vi "Attach Node.vi"(0 "TREE in":refnum<class "MyTreeAPI.lvclass">, 5 "Parent Node":string, 7 "Node ID":string, 9 "Node Name":string, 11 "error in (no error)":errorcluster, 12 "Symbol Index":i32) -> (4 "TREE out":refnum<class "MyTreeAPI.lvclass">, 6 "Node ID":string, 15 "error out":errorcluster)   [LabVIEW 2015, in "MyTreeAPI.lvclass"]
uses:
  MyTreeAPI.lvclass
  MyTreeAPI.lvclass/MyTreeAPI.ctl
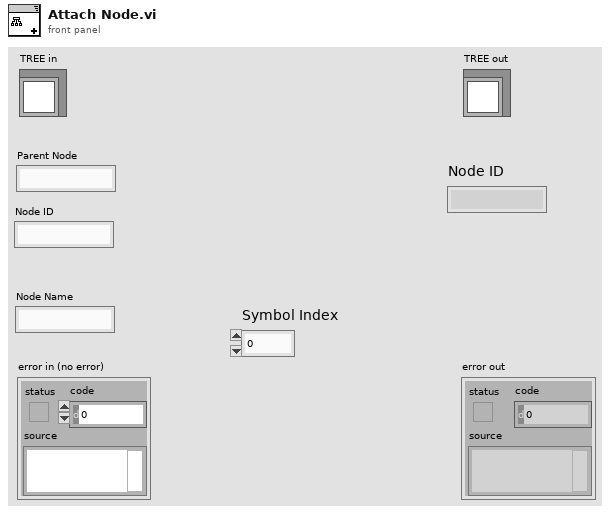
[diagram p1: front panel]
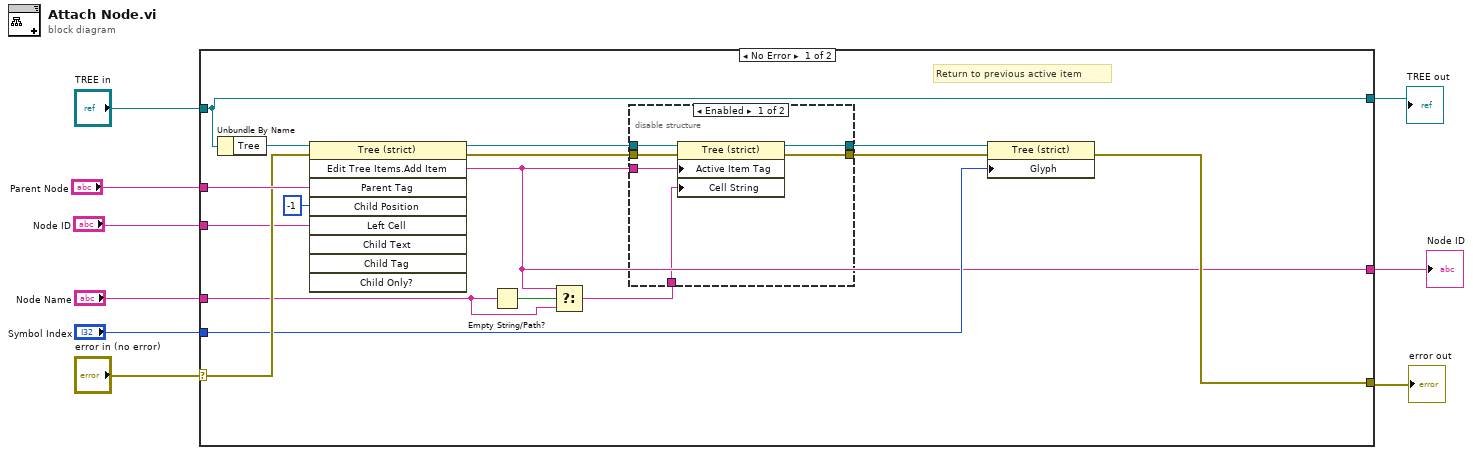
[diagram p0: block diagram]
diagram:
  n1 = case shown="No Error" "error in (no error)" {
    selector: "error in (no error)" -> [w21 w35]
    tunnel: [w19 w35] -> w8
    tunnel: [w25 w34] -> w6
    tunnel: "TREE in" -> [w25 w34]
    tunnel: "Parent Node" -> [w22 _]
    tunnel: "Symbol Index" -> [w20 _]
    tunnel: "Node ID" -> [w18 _]
    tunnel: "Node Name" -> [w13 _]
    tunnel: [w14 _] -> w1
    frame No Error {
      # "Return to previous active item"
      n2 = Unbundle By Name(w25) -> ("Tree"=w23:refnum<vi>)
      n3 = invoke class="Tree (strict)" method="Edit Tree Items.Add Item"(reference=w23, error in=w21, "Parent Tag"=w22, "Child Position"=-1, "Left Cell"=w18) -> (reference out=w17:refnum<vi>, error out=w16:errorcluster, "Edit Tree Items:Add Item"=w14:string)  [unwired: 4 in, 6 out]
      n4 = Empty String/Path?(string/path=w13) -> (empty?=w15:bool)
      n5 = Select(t=w14, s=w15, f=w13) -> (s? t:f=w12:string)
      n6 = disable-structure shown="Enabled" {
        disable-tunnel: w17 -> [w29 w33]
        disable-tunnel: w16 -> [w28 w32]
        disable-tunnel: [w31 w33] -> w11
        disable-tunnel: [w30 w32] -> w10
        disable-tunnel: w14 -> [w27 _]
        disable-tunnel: w12 -> [w26 _]
        frame Enabled {
          n7 = property class="Tree (strict)"(reference=w29, error in=w28, "Active Item Tag"=w27, "Cell String"=w26) -> (reference out=w31:refnum<vi>, error out=w30:errorcluster)
        }
        frame Disabled {
        }
      }
      n8 = property class="Tree (strict)"(reference=w11, error in=w10, "Glyph"=w20) -> (error out=w19:errorcluster)  [unwired: 1 out]
    }
    frame Error {
    }
  }
  "error out" <- w8
  "TREE out" <- w6
  "Node ID" <- w1
